vi "Simulated IO For Digital Pattern Generator.vi"(0 "sim I/O info in":T1, 9 "data from node input terminals":variant[](array[variant]), 11 "input from node terminal error in":errorcluster) -> (4 "sim I/O info out":T1, 10 "data to node output terminals":variant[](array[variant]), 15 "output to node terminal error out":errorcluster)   [LabVIEW 2016]
uses:
  <vilib>/FPGA/viExecutionOnDevComputer/simIO/customVI/Sim IO Info.ctl
  <vilib>/rvi/customViForEmulation/niLvFPGAUserSpecifiedEmulationVISupport.lvclass
  Host/Typedefs/IO Buffer Operation.ctl
  <vilib>/FPGA/viExecutionOnDevComputer/simIO/customVI/niFPGA Simulated IO.lvlib
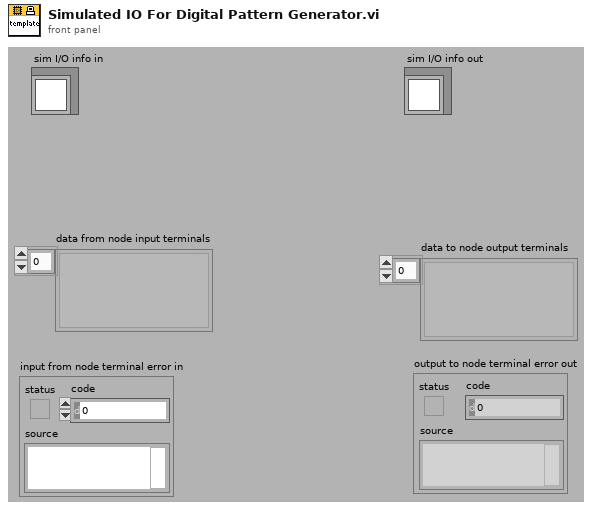
[diagram p1: front panel]
types:
  T1 = typedef "niFPGA Simulated IO.lvlib/Sim IO Info.ctl" = refnum<class "niLvFPGAUserSpecifiedEmulationVISupport.lvclass">
  T2 = typedef "niFPGA Simulated IO.lvlib/Execution Stage.ctl" = enum16{"Initializing", "Running", "Shutting Down"}
  T3 = typedef "IO Buffer Operation.ctl" = enum16{"Initialize", "Write IO Data_Rd", "Read IO Data_Rd", "Write IO Data_Wr", "Read IO Data_Wr", "Write  IO Data_Dir", "Read  IO Data_Dir", "Write Host to Target FIFO", "Read Host to Target FIFO", "Write Target to Host FIFO", "Read Target to Host FIFO", "Write Monitor Enable?", "Read Monitor Enable?", "Close"}
  T4 = typedef "niFPGA Simulated IO.lvlib/Node or Element Type.ctl" = enum16{"Read I/O", "Write I/O", "Method", "Read Property", "Write Property"}
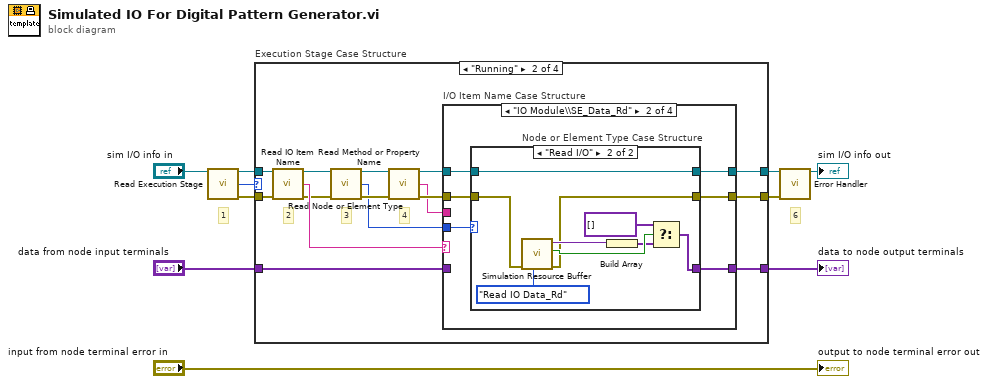
[diagram p0: block diagram]
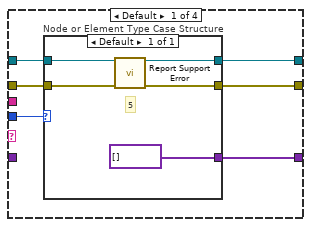
[diagram p3: hidden frame]
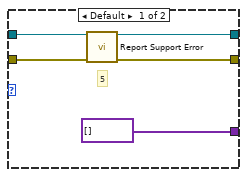
[diagram p4: hidden frame]
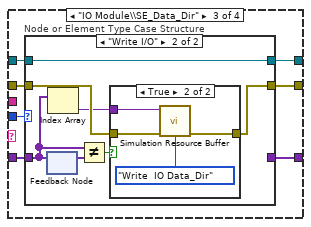
[diagram p5: hidden frame]
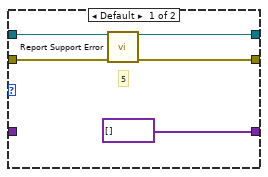
[diagram p6: hidden frame]
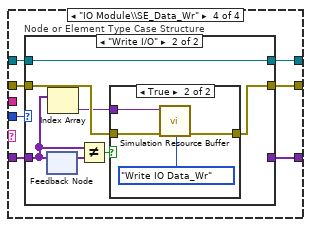
[diagram p8: hidden frame]
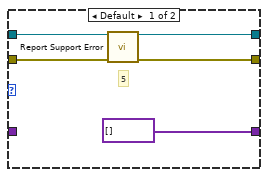
[diagram p9: hidden frame]
diagram:
  # "1"
  # "6"
  n1 = call <vilib>:"Read Execution Stage.vi"("sim I/O info in"="sim I/O info in") -> ("sim I/O info out"=w3:T1, "execution stage"=w1:T2, "error out"=w2:errorcluster)  [unwired: 1 in, 11 out]
  n2 = case "Execution Stage Case Structure" shown="\"Running\"" w1 {
    tunnel: [_ w26 _ _] -> w9
    tunnel: [w12 w21 w108 w110] -> w4
    tunnel: [w11 w17 w107 w109] -> w6
    tunnel: w3 -> [w11 w15 w107 w109]
    tunnel: w2 -> [w12 w14 w108 w110]
    tunnel: "data from node input terminals" -> [_ w27 _ _]
    frame "Initializing" {
    }
    frame "Running" {
      # "4"
      # "3"
      # "2"
      n3 = call <vilib>:"Read IO Item Name.vi"("sim I/O info in"=w15, "error in (no error)"=w14) -> ("sim I/O info out"=w16:T1, "I/O item name"=w25:string, "error out"=w24:errorcluster)  [unwired: 11 out]
      n4 = call <vilib>:"Read Node or Element Type.vi"("sim I/O info in"=w16, "error in (no error)"=w24) -> ("sim I/O info out"=w13:T1, "node or element type"=w22:T4, "error out"=w23:errorcluster)  [unwired: 11 out]
      n5 = call <vilib>:"Read Method or Property Name.vi"("sim I/O info in"=w13, "error in (no error)"=w23) -> ("sim I/O info out"=w19:T1, "method or property name"=w18:string, "error out"=w20:errorcluster)  [unwired: 11 out]
      n6 = case "I/O Item Name Case Structure" shown="\"IO Module\\\\SE_Data_Rd\"" w25 {
        tunnel: w27 -> [_ _ w59 w83]
        tunnel: [w29 w40 w61 w85] -> w26
        tunnel: w20 -> [w33 w44 w65 w89]
        tunnel: [w32 w43 w64 w88] -> w21
        tunnel: w19 -> [w31 w42 w63 w87]
        tunnel: [w30 w41 w62 w86] -> w17
        tunnel: w22 -> [w28 w39 w60 w84]
        tunnel: w18 -> [_ _ _ _]
        frame Default {
          n7 = case "Node or Element Type Case Structure" shown="Default" w28 {
            tunnel: w33 -> [w38]
            tunnel: [w37] -> w32
            tunnel: w31 -> [w36]
            tunnel: [w35] -> w30
            tunnel: [variant[] []] -> w29
            frame Default {
              # "5"
              n8 = call <vilib>:"Report Support Error.vi"("sim I/O info in"=w36, "error in (no error)"=w38) -> ("sim I/O info out"=w35:T1, "error out"=w37:errorcluster)  [unwired: 12 out]
            }
          }
        }
        frame "IO Module\\SE_Data_Rd" {
          n9 = case "Node or Element Type Case Structure" shown="\"Read I/O\"" w39 {
            tunnel: w44 -> [w49 w52]
            tunnel: [w48 w51] -> w43
            tunnel: w42 -> [w47 w50]
            tunnel: [w46 w50] -> w41
            tunnel: [variant[] [] w53] -> w40
            frame Default {
              # "5"
              n10 = call <vilib>:"Report Support Error.vi"("sim I/O info in"=w47, "error in (no error)"=w49) -> ("sim I/O info out"=w46:T1, "error out"=w48:errorcluster)  [unwired: 12 out]
            }
            frame "Read I/O" {
              n11 = call "Simulation Resource Buffer.vi"("IO Buffer Operation"=IO_Buffer_Operation."Read IO Data_Rd", "error in (no error)"=w52) -> ("error out"=w51:errorcluster, "Timed Out?"=w57:bool, "Data out"=w56:variant)  [unwired: 7 in]
              n12 = Build Array(w56) -> (w55:variant[])
              n13 = Select(t=variant[] [], s=w57, f=w55) -> (s? t:f=w53:variant[])
            }
          }
        }
        frame "IO Module\\SE_Data_Dir" {
          n14 = case "Node or Element Type Case Structure" shown="\"Write I/O\"" w60 {
            tunnel: w65 -> [w70 w77]
            tunnel: [w69 w76] -> w64
            tunnel: w63 -> [w68 w75]
            tunnel: [w67 w75] -> w62
            tunnel: [variant[] [] _] -> w61
            tunnel: w59 -> [_ w72]
            frame Default {
              # "5"
              n15 = call <vilib>:"Report Support Error.vi"("sim I/O info in"=w68, "error in (no error)"=w70) -> ("sim I/O info out"=w67:T1, "error out"=w69:errorcluster)  [unwired: 12 out]
            }
            frame "Write I/O" {
              n16 = feedback-in #1(w72) -> ()
              n17 = feedback #1() -> (w74:variant[])  [unwired: 1 in]
              n18 = Index Array(array=w72) -> (element=w71:variant)  [unwired: 1 in]
              n19 = Not Equal?(x=w72, y=w74) -> (x != y?=w73:bool)
              n20 = case shown="True" w73 {
                tunnel: w77 -> [w78 w81]
                tunnel: [w78 w80] -> w76
                tunnel: w71 -> [_ w79]
                frame False {
                }
                frame True {
                  n21 = call "Simulation Resource Buffer.vi"("IO Buffer Operation"=IO_Buffer_Operation."Write  IO Data_Dir", "error in (no error)"=w81, "Data in"=w79) -> ("error out"=w80:errorcluster)  [unwired: 6 in, 2 out]
                }
              }
            }
          }
        }
        frame "IO Module\\SE_Data_Wr" {
          n22 = case "Node or Element Type Case Structure" shown="\"Write I/O\"" w84 {
            tunnel: w89 -> [w94 w101]
            tunnel: [w93 w100] -> w88
            tunnel: w87 -> [w92 w99]
            tunnel: [w91 w99] -> w86
            tunnel: [variant[] [] _] -> w85
            tunnel: w83 -> [_ w96]
            frame Default {
              # "5"
              n23 = call <vilib>:"Report Support Error.vi"("sim I/O info in"=w92, "error in (no error)"=w94) -> ("sim I/O info out"=w91:T1, "error out"=w93:errorcluster)  [unwired: 12 out]
            }
            frame "Write I/O" {
              n24 = feedback-in #2(w96) -> ()
              n25 = feedback #2() -> (w98:variant[])  [unwired: 1 in]
              n26 = Index Array(array=w96) -> (element=w95:variant)  [unwired: 1 in]
              n27 = Not Equal?(x=w96, y=w98) -> (x != y?=w97:bool)
              n28 = case shown="True" w97 {
                tunnel: w101 -> [w102 w105]
                tunnel: [w102 w104] -> w100
                tunnel: w95 -> [_ w103]
                frame False {
                }
                frame True {
                  n29 = call "Simulation Resource Buffer.vi"("IO Buffer Operation"=IO_Buffer_Operation."Write IO Data_Wr", "error in (no error)"=w105, "Data in"=w103) -> ("error out"=w104:errorcluster)  [unwired: 6 in, 2 out]
                }
              }
            }
          }
        }
      }
    }
    frame "Shutting Down" {
    }
    frame Default {
    }
  }
  "data to node output terminals" <- w9
  n30 = call <vilib>:"Error Handler.vi"("sim I/O info in"=w6, "error in"=w4) -> ("sim I/O info out"=→"sim I/O info out":T1)  [unwired: 13 out]
  "output to node terminal error out" <- "input from node terminal error in"
